vi "TC_E_VtoC.vi"(11 "Thermocouple Voltage":dbl caption="热电偶电压" format="%0.6f") -> (3 "T(c)":dbl format="%#_16f")   [LabVIEW 2012]
doc: "功能：\n\nB型热电偶电压转换为摄氏度。\n\ncsxcs_366创建。"
uses:
  <vilib>/Analysis/polynomials.llb/Scalar Polynomial Evaluation (DBL).vi
  <vilib>/Analysis/NI_AALPro.lvlib
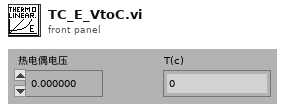
[diagram p1: front panel]
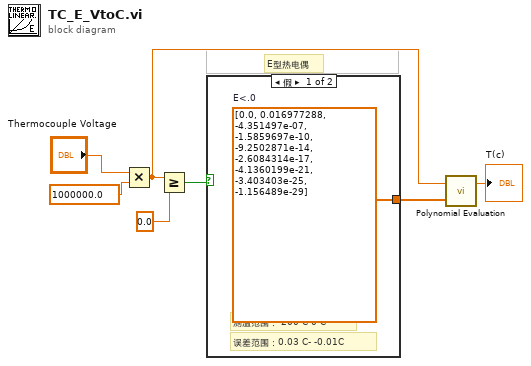
[diagram p0: block diagram]
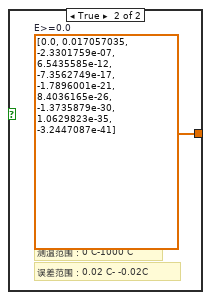
[diagram p2: hidden frame]
diagram:
  # "E型热电偶"
  n1 = Multiply(x="Thermocouple Voltage", y=1000000.0) -> (x*y=w3:dbl)
  n2 = Greater Or Equal?(x=w3, y=0.0) -> (x >= y?=w4:bool)
  n3 = case shown="假" w4 {
    tunnel: [w8 w9] -> w1
    frame False {
      w8 = dbl[] [0.0, 0.016977288, -4.351497e-07, -1.5859697e-10, -9.2502871e-14, -2.6084314e-17, -4.1360199e-21, -3.403403e-25, -1.156489e-29]  # E<.0
      # "误差范围：0.03 C- -0.01C"
      # "测温范围：-200 C-0 C"
    }
    frame True {
      w9 = dbl[] [0.0, 0.017057035, -2.3301759e-07, 6.5435585e-12, -7.3562749e-17, -1.7896001e-21, 8.4036165e-26, -1.3735879e-30, 1.0629823e-35, -3.2447087e-41]  # E>=0.0
      # "误差范围：0.02 C- -0.02C"
      # "测温范围：0 C-1000 C"
    }
  }
  n4 = call-poly <vilib>:"Polynomial Evaluation.vi"("P(x)"=w1, "a"=w3) -> ("P(a)"=→"T(c)":dbl)  [unwired: 1 out]
